vi "tarea.vi"() -> ()   [LabVIEW 2020]
panel:
  in  "Boolean":bool
  in  "restar":dbl
  in  "sumar":i32
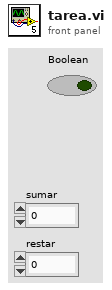
[diagram p1: front panel]
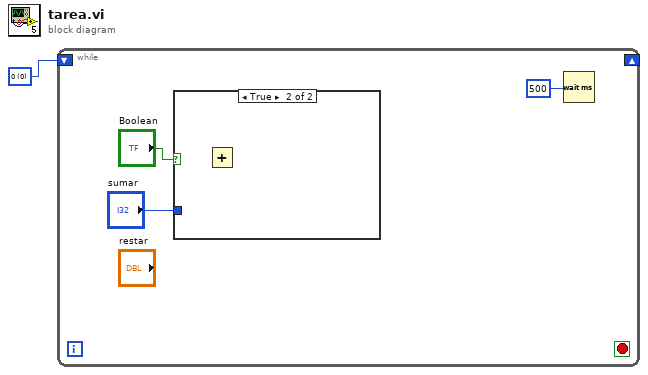
[diagram p0: block diagram]
diagram:
  w1 = u16 0 items=["0"]
  n1 = while {
    shift-right: _ -> [w5]
    shift-left: w1 -> [w7]
    stop <- w4 stop-if-true
    n2 = case shown="True" "Boolean" {
      tunnel: "sumar" -> [_ _]
      frame False {
      }
      frame True {
        n3 = Add() -> ()  [unwired: 2 in, 1 out]
      }
    }
    n4 = Wait (ms)(milliseconds to wait=500) -> ()  [unwired: 1 out]
  }
